vi "Aborts-Loop.vi"(0 "Message Queues":T1, 1 "Processed Data Notifier":refnum<notifier>, 3 "error in":errorcluster) -> (10 "error out":errorcluster)   [LabVIEW 2024]
uses:
  support/Message Queue/All Message Queues.ctl
  support/Message Queue/Message Cluster.ctl
  support/Control/Array Data Constant.ctl
  Abort State.ctl
  Abort Parameters.ctl
  Configuration/Calibration Configuration.ctl
  <vilib>/Utility/error.llb/Error Cluster From Error Code.vi
  <vilib>/ErrorRing/Error Ring.xnode
  support/Message Queue/Message Queue.lvlib
panel:
  out "Loop-5 Iteration Counter":i32
  out "Loop-5 Iteration Clock (ms)":u32
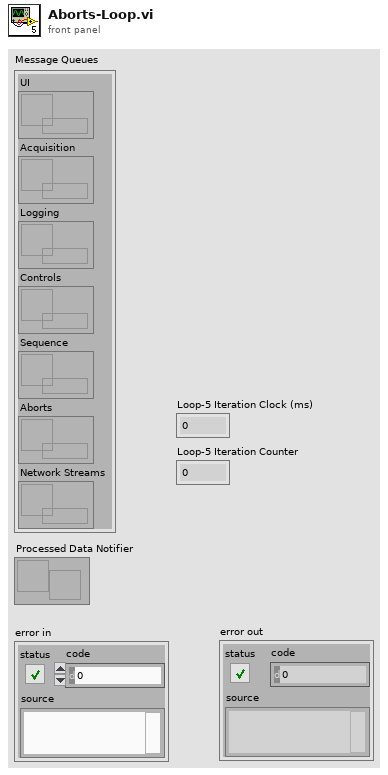
[diagram p1: front panel]
types:
  T1 = typedef "Message Queue.lvlib/All Message Queues.ctl" = cluster{"UI":refnum<queue>, "Acquisition":refnum<queue>, "Logging":refnum<queue>, "Controls":refnum<queue>, "Sequence":refnum<queue>, "Aborts":refnum<queue>, "Network Streams":refnum<queue>}
  T2 = typedef "Calibration Configuration.ctl" = cluster{"ai Calibration Slope":dbl[], "ai Calibration Offset":dbl[], "ai Sensor Names ":string[], "tc Sensor Names":string[], "di Sensor Names":string[], "do Sensor Names":string[], "bc Sensor Names":string[], "ai Sensor Units":string[], "tc Sensor Units":string[], "bc Sensor Units":string[]}
  T3 = typedef "Abort Parameters.ctl" = cluster{"Sequence Delay (s)":dbl, "Sequence Duration (s)":dbl, "Abort Criteria":cluster{"Channel Name\n":enum16{"[0]", "[1]", "[2]", "[3]", "[4]", "[5]", "[6]", "[7]", "[8]", "[9]", "[10]", "[11]", "[12]", "[13]", "[14]", "[15]", "[16]", "[17]", "[18]", "[19]", "[20]", "[21]", "[22]", "[23]", "[24]", "[25]", "[26]", "[27]", "[28]", "[29]", "[30]", "[31]", "[32]", "[33]", "[34]", "[35]", "[36]", "[37]", "[38]", "[39]", "[40]", "[41]", "[42]", "[43]", "[44]", "[45]", "[46]", "[47]", "[48]", "[49]"}, "Comparison\n":u16, "Threshold":dbl, "Time on (s)":dbl, "Time off (s)":dbl, "Enabled":bool}[]}
  T4 = typedef "Abort State.ctl" = enum16{"Idle", "Checking", "Reset"}
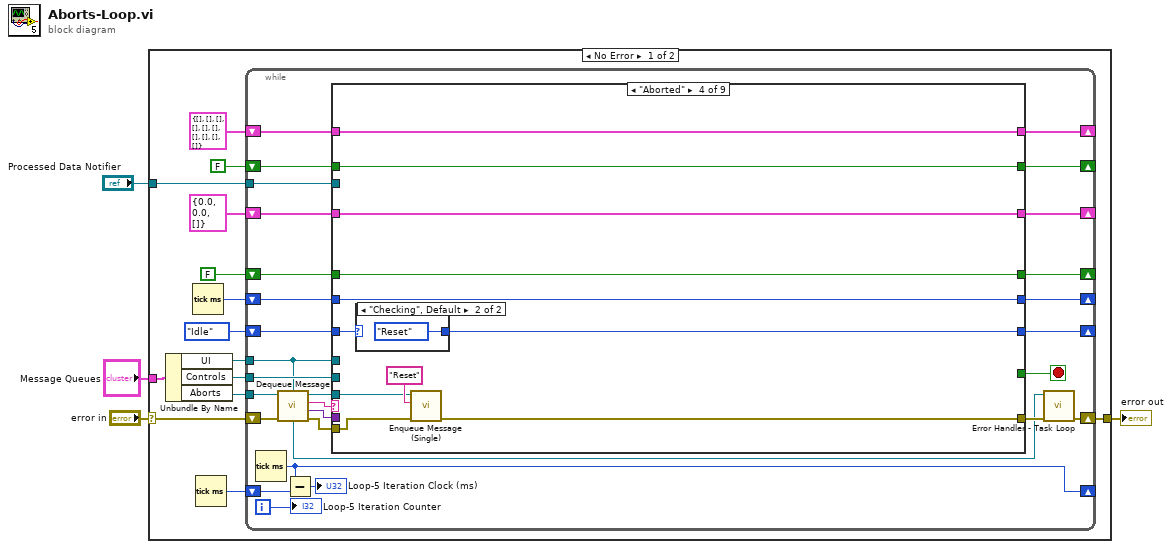
[diagram p0: block diagram]
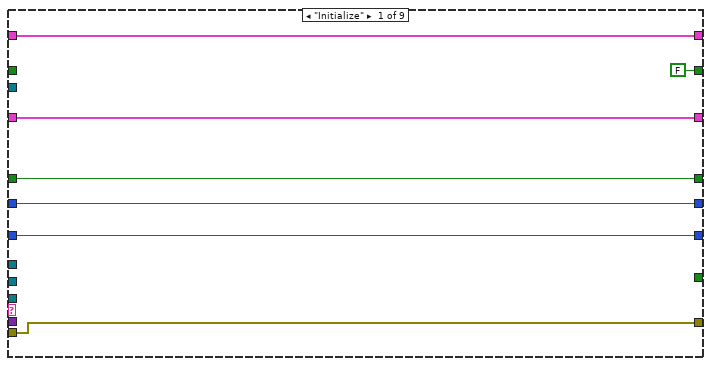
[diagram p2: hidden frame]
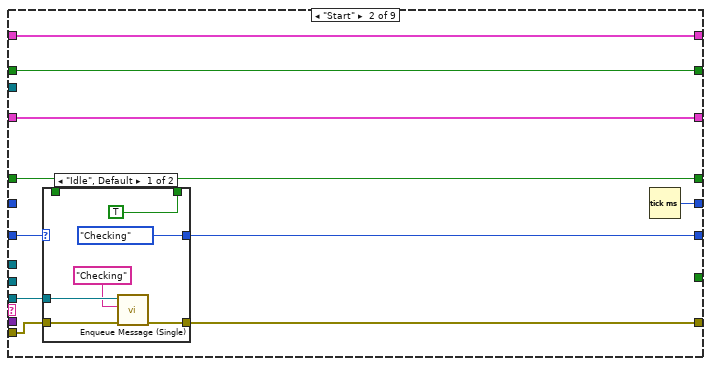
[diagram p3: hidden frame]
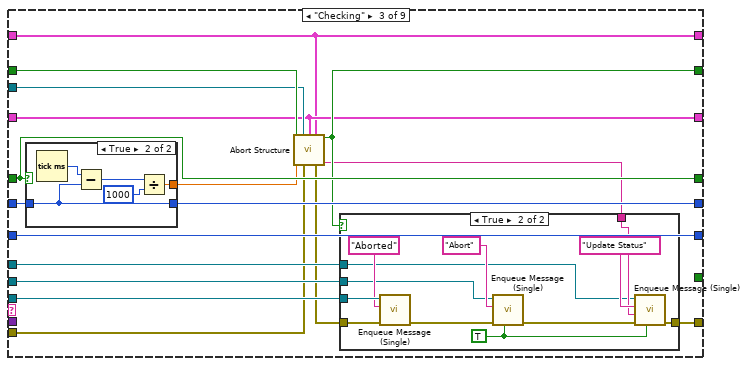
[diagram p5: hidden frame]
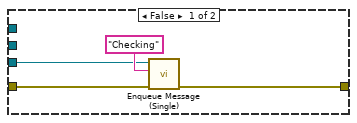
[diagram p6: hidden frame]
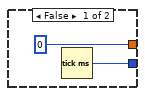
[diagram p7: hidden frame]
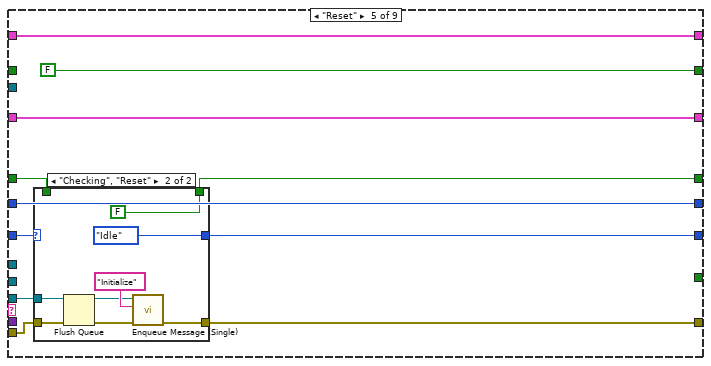
[diagram p9: hidden frame]
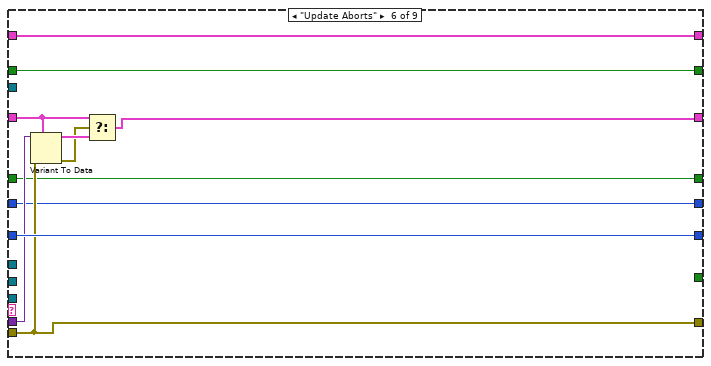
[diagram p11: hidden frame]
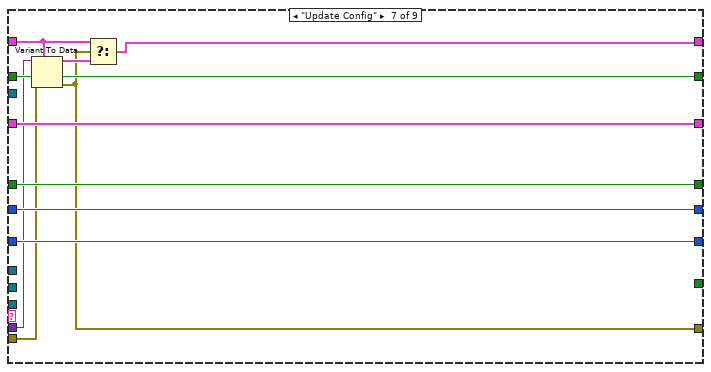
[diagram p12: hidden frame]
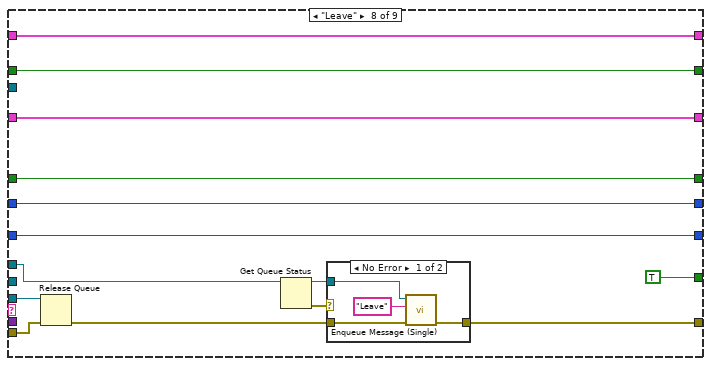
[diagram p13: hidden frame]
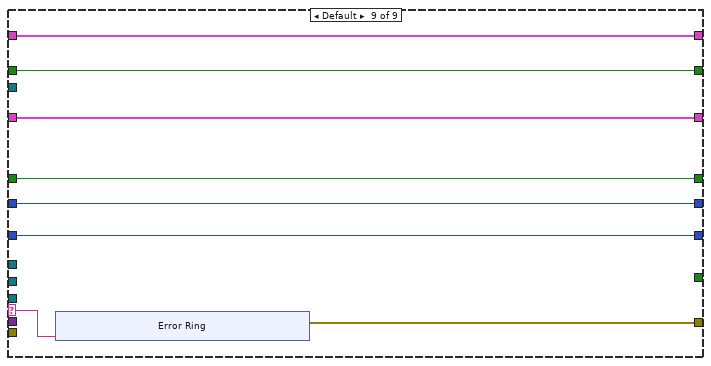
[diagram p15: hidden frame]
diagram:
  n1 = case shown="No Error" "error in" {
    selector: "error in" -> [w18 w205]
    tunnel: [w17 w205] -> w3
    tunnel: "Message Queues" -> [w16 _]
    tunnel: "Processed Data Notifier" -> [w11 _]
    frame No Error {
      n2 = Unbundle By Name(w16) -> ("UI"=w13:refnum<queue>, "Controls"=w15:refnum<queue>, "Aborts"=w14:refnum<queue>)
      n3 = Tick Count (ms)() -> (millisecond timer value=w9:u32)
      n4 = Tick Count (ms)() -> (millisecond timer value=w6:u32)
      n5 = while {
        shift-right: [w39] -> w17
        shift-left: w18 -> [w45]
        tunnel: w15 -> [w38]
        tunnel: w14 -> [w46]
        tunnel: w13 -> [w27]
        shift-right: [w36] -> _
        shift-left: Abort_State."Idle" ("Abort State") -> [w37]
        tunnel: w11 -> [w35]
        shift-right: [w33] -> _
        shift-left: T3 {"Sequence Delay (s)"=0.0, "Sequence Duration (s)"=0.0, "Abort Criteria"=[]} ("Abort Parameters") -> [w34]
        shift-right: [w30] -> _
        shift-left: FALSE -> [w31]
        shift-right: [w28] -> _
        shift-left: w9 -> [w29]
        shift-right: [w25] -> _
        shift-left: FALSE -> [w26]
        shift-right: [w22] -> _
        shift-left: w6 -> [w23]
        shift-right: [w20] -> _
        shift-left: T2 {"ai Calibration Slope"=[], "ai Calibration Offset"=[], "ai Sensor Names "=[], "tc Sensor Names"=[], "di Sensor Names"=[], "do Sensor Names"=[], "bc Sensor Names"=[], "ai Sensor Units"=[], "tc Sensor Units"=[], "bc Sensor Units"=[]} ("Calibration Configuration") -> [w19]
        i -> [w21]
        stop <- w32 stop-if-true
        n6 = Tick Count (ms)() -> (millisecond timer value=w22:u32)
        n7 = call "Dequeue Message.vi"("error in (no error)"=w45, "Message Queue"=w46) -> ("error out"=w41:errorcluster, "Message Data"=w42:variant, "Message"=w43:string, "dup Message Queue"=w44:refnum<queue>)  [unwired: 6 in]
        n8 = Subtract(x=w22, y=w23) -> (x-y=→"Loop-5 Iteration Clock (ms)":u32)
        n9 = case shown="\"Aborted\"" w43 {
          selector: w43 -> [_ _ _ _ _ _ _ _ w197]
          tunnel: w44 -> [_ w62 w84 w116 w135 _ _ w183 _]
          tunnel: w42 -> [_ _ _ _ _ w157 w163 _ _]
          tunnel: w41 -> [w53 w61 w78 w115 w134 w153 w162 w184 _]
          tunnel: [w53 w60 w74 w114 w133 w153 w160 w175 w196] -> w40
          tunnel: w38 -> [_ _ w86 _ _ _ _ _ _]
          tunnel: w27 -> [_ _ w85 _ _ _ _ w171 _]
          tunnel: w37 -> [w52 w64 w90 w122 w137 w159 w166 w181 w195]
          tunnel: [w52 w63 w90 w121 w136 w159 w166 w181 w195] -> w36
          tunnel: w35 -> [_ _ w81 _ _ _ _ _ _]
          tunnel: w34 -> [w51 w59 w80 w124 w132 w156 w169 w182 w194]
          tunnel: [w51 w59 w80 w124 w132 w155 w169 w182 w194] -> w33
          tunnel: [_ _ _ _ _ _ _ TRUE _] -> w32
          tunnel: w31 -> [w50 w57 w87 w123 w129 w152 w168 w180 w193]
          tunnel: [w50 w58 w87 w123 w131 w152 w168 w180 w193] -> w30
          tunnel: w29 -> [w49 _ w89 w118 w130 w151 w167 w179 w192]
          tunnel: [w49 w54 w88 w118 w130 w151 w167 w179 w192] -> w28
          tunnel: w26 -> [_ w56 w83 w120 _ w150 w170 w178 w191]
          tunnel: [FALSE ("Abort Constant Out") w56 w82 w120 FALSE w150 w170 w178 w191] -> w25
          tunnel: [w48 w55 w75 w119 w127 w149 w161 w174 w190] -> w20
          tunnel: w19 -> [w48 w55 w75 w119 w127 w149 w164 w174 w190]
          frame "Initialize" {
          }
          frame "Start" {
            n10 = case shown="\"Idle\", Default" w64 {
              selector: w64 -> [_ w73]
              tunnel: [Abort_State."Checking" ("Abort State") w73] -> w63
              tunnel: w62 -> [w67 _]
              tunnel: w61 -> [w68 w72]
              tunnel: [w69 w72] -> w60
              tunnel: [TRUE w71] -> w58
              tunnel: w57 -> [_ w71]
              frame "Idle", Default {
                n11 = call "Enqueue Message (Single).vi"("error in (no error)"=w68, "Message"="Checking", "Message Queue"=w67) -> ("error out"=w69:errorcluster)  [unwired: 7 in, 1 out]
              }
              frame "Checking" {
              }
            }
            n12 = Tick Count (ms)() -> (millisecond timer value=w54:u32)
          }
          frame "Checking" {
            n13 = case shown="True" w87 {
              tunnel: w89 -> [_ w110]
              tunnel: [0 w109] -> w79
              tunnel: [w107 w110] -> w88
              frame False {
                n14 = Tick Count (ms)() -> (millisecond timer value=w107:u32)
              }
              frame True {
                n15 = Tick Count (ms)() -> (millisecond timer value=w112:u32)
                n16 = Subtract(x=w112, y=w110) -> (x-y=w111:u32)
                n17 = Divide(x=w111, y=1000) -> (x/y=w109:dbl)
              }
            }
            n18 = call "Abort Structure.vi"("Abort Constant In"=w83, "Processed Data Notifier"=w81, "Abort Parameters"=w80, "Calibration Configuration"=w75, "Clock timer (s)"=w79, "error in"=w78) -> ("Abort Constant Out"=w82:bool, "error out"=w77:errorcluster, "Status"=w76:string)  [unwired: 7 in]
            n19 = case shown="True" w82 {
              tunnel: w77 -> [w92 w105]
              tunnel: [w91 w102] -> w74
              tunnel: w86 -> [_ w99]
              tunnel: w84 -> [w93 w104]
              tunnel: w85 -> [_ w97]
              tunnel: w76 -> [_ w100]
              frame False {
                n20 = call "Enqueue Message (Single).vi"("error in (no error)"=w92, "Message"="Checking", "Message Queue"=w93) -> ("error out"=w91:errorcluster)  [unwired: 7 in, 1 out]
              }
              frame True {
                w95 = TRUE ("Priority Message? (F)")
                n21 = call "Enqueue Message (Single).vi"("error in (no error)"=w105, "Message"="Aborted", "Message Queue"=w104) -> ("error out"=w98:errorcluster)  [unwired: 7 in, 1 out]
                n22 = call "Enqueue Message (Single).vi"("Priority Message? (F)"=w95, "error in (no error)"=w98, "Message"="Abort", "Message Queue"=w99) -> ("error out"=w96:errorcluster)  [unwired: 6 in, 1 out]
                n23 = call "Enqueue Message (Single).vi"("Priority Message? (F)"=w95, "error in (no error)"=w96, "Message Data"=w100, "Message"="Update Status", "Message Queue"=w97) -> ("error out"=w102:errorcluster)  [unwired: 5 in, 1 out]
              }
            }
          }
          frame "Aborted" {
            n24 = case shown="\"Checking\", Default" w122 {
              selector: w122 -> [w125 _]
              tunnel: [w125 Abort_State."Reset" ("Abort State")] -> w121
              frame "Reset" {
              }
              frame "Checking", Default {
              }
            }
            n25 = call "Enqueue Message (Single).vi"("error in (no error)"=w115, "Message"="Reset", "Message Queue"=w116) -> ("error out"=w114:errorcluster)  [unwired: 7 in, 1 out]
          }
          frame "Reset" {
            n26 = case shown="\"Checking\", \"Reset\"" w137 {
              selector: w137 -> [w140 _]
              tunnel: [w140 Abort_State."Idle" ("Abort State")] -> w136
              tunnel: w135 -> [_ w143]
              tunnel: w134 -> [w139 w144]
              tunnel: [w139 w147] -> w133
              tunnel: [w138 FALSE] -> w131
              tunnel: w129 -> [w138 _]
              frame "Idle" {
              }
              frame "Checking", "Reset" {
                n27 = Flush Queue(queue=w143, error in (no error)=w144) -> (queue out=w142:refnum<queue>, error out=w141:errorcluster)  [unwired: 1 out]
                n28 = call "Enqueue Message (Single).vi"("error in (no error)"=w141, "Message"="Initialize", "Message Queue"=w142) -> ("error out"=w147:errorcluster)  [unwired: 7 in, 1 out]
              }
            }
          }
          frame "Update Aborts" {
            n29 = Variant To Data(error in=w153, type=w156, Variant=w157) -> (data=w158:T3, error out=w154:errorcluster)
            n30 = Select(t=w156, s=w154, f=w158) -> (s? t:f=w155:T3)
          }
          frame "Update Config" {
            n31 = Variant To Data(error in=w162, type=w164, Variant=w163) -> (data=w165:T2, error out=w160:errorcluster)
            n32 = Select(t=w164, s=w160, f=w165) -> (s? t:f=w161:T2)
          }
          frame "Leave" {
            n33 = Release Queue(queue=w183, error in (no error)=w184) -> (error out=w176:errorcluster)  [unwired: 1 in, 2 out]
            n34 = Get Queue Status(queue=w171) -> (queue out=w173:refnum<queue>, error out=w172:errorcluster)  [unwired: 2 in, 6 out]
            n35 = case shown="No Error" w172 {
              tunnel: w176 -> [w187 w189]
              tunnel: [w186 w189] -> w175
              tunnel: w173 -> [w185 _]
              frame No Error {
                n36 = call "Enqueue Message (Single).vi"("error in (no error)"=w187, "Message"="Leave", "Message Queue"=w185) -> ("error out"=w186:errorcluster)  [unwired: 7 in, 1 out]
              }
              frame Error {
              }
            }
          }
          frame Default {
            n37 = xnode "Error Ring"("parameter 0"=w197) -> ("error out"=w196:errorcluster)
          }
        }
        n38 = call "Error Handler - Task Loop.vi"("error in (no error)"=w40, "Message Queue"=w27) -> ("dup error in"=w39:errorcluster)  [unwired: 8 in, 1 out]
        "Loop-5 Iteration Counter" <- w21
      }
    }
    frame Error {
    }
  }
  "error out" <- w3
